vi "Image to VI Icons.vi"   [LabVIEW 2015]
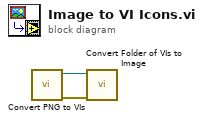
[diagram p0: block diagram]
diagram:
  n1 = call <resource>:"Convert PNG to VIs.vi"() -> ("error out"=w2:errorcluster, "directory copy"=w1:path)  [unwired: 10 in]
  n2 = call <resource>:"Convert Folder of VIs to Image.vi"("error in (no error)"=w2, "Folder Path"=w1) -> ()  [unwired: 9 in, 1 out]
